vi "Insight_Marquee_Progress.vi"(11 "x":u8) -> (0 "Progress Indicator":cluster{u8, u8}(slide)={0, 49} scale=0.0..100.0, 3 "x (out)":u8)   [LabVIEW 2014]
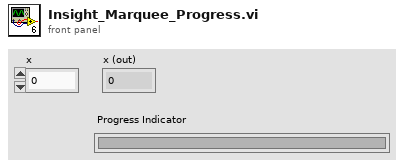
[diagram p1: front panel]
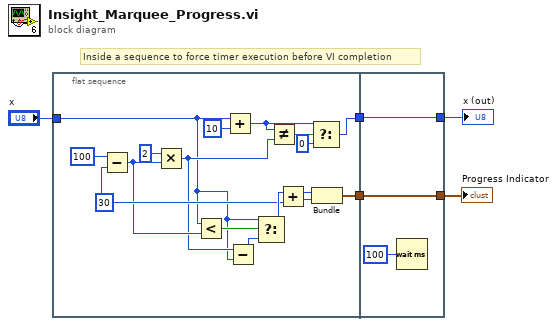
[diagram p0: block diagram]
diagram:
  # "Inside a sequence to force timer execution before VI completion"
  n1 = flat-sequence {
    tunnel: "x" -> [w7]
    tunnel: [w6] -> w2
    tunnel: [w17] -> w1
    tunnel: [w23] -> w4
    tunnel: [w24] -> w5
    tunnel: w2 -> [w24]
    tunnel: w1 -> [w23]
    frame #0 {
      w12 = u8 30 ("Search Indicator 2")
      n2 = Subtract(x=u8 100 ("Search Indicator 2"), y=w12) -> (x-y=w9:u8)
      n3 = Multiply(x=u8 2, y=w9) -> (x*y=w8:u8)
      n4 = Less?(x=w7, y=w9) -> (x < y?=w14:bool)
      n5 = Add(x=w7, y=u8 10) -> (x+y=w18:u8)
      n6 = Subtract(x=w8, y=w7) -> (x-y=w10:u8)
      n7 = Select(t=w7, s=w14, f=w10) -> (s? t:f=w13:u8)
      n8 = Not Equal?(x=w18, y=w8) -> (x != y?=w19:bool)
      n9 = Add(x=w13, y=w12) -> (x+y=w21:u8)
      n10 = Select(t=w18, s=w19, f=u8 0) -> (s? t:f=w17:u8)
      n11 = Bundle("x"=w13, w21) -> (w6:cluster{"x":u8, u8})  [unwired: 1 in]
    }
    frame #1 {
      n12 = Wait (ms)(milliseconds to wait=u32 100) -> ()  [unwired: 1 out]
    }
  }
  "Progress Indicator" <- w5
  "x (out)" <- w4
